vi "Open.vi"(8 "Error In":errorcluster, 10 "Enable Gestures? (T)":bool=TRUE) -> (0 "Error Out":errorcluster, 3 "Leap Handle":T1)   [LabVIEW 2014]
uses:
  Typedef 2.0/Leap Handle.ctl
  C:/Users/Frax/Desktop/Progetti avanzati Labview/Smart Wristband/Smart Wristband/Leap Motion VIs 2.0/LeapCSharp.NET4.0.dll
  LeapCSharp.NET4.0.dll
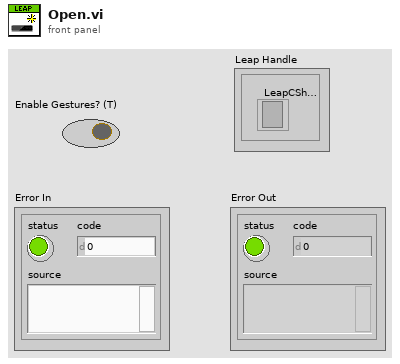
[diagram p1: front panel]
types:
  T1 = typedef "Leap Handle.ctl" = cluster{"LeapCSharp":refnum<k24>}
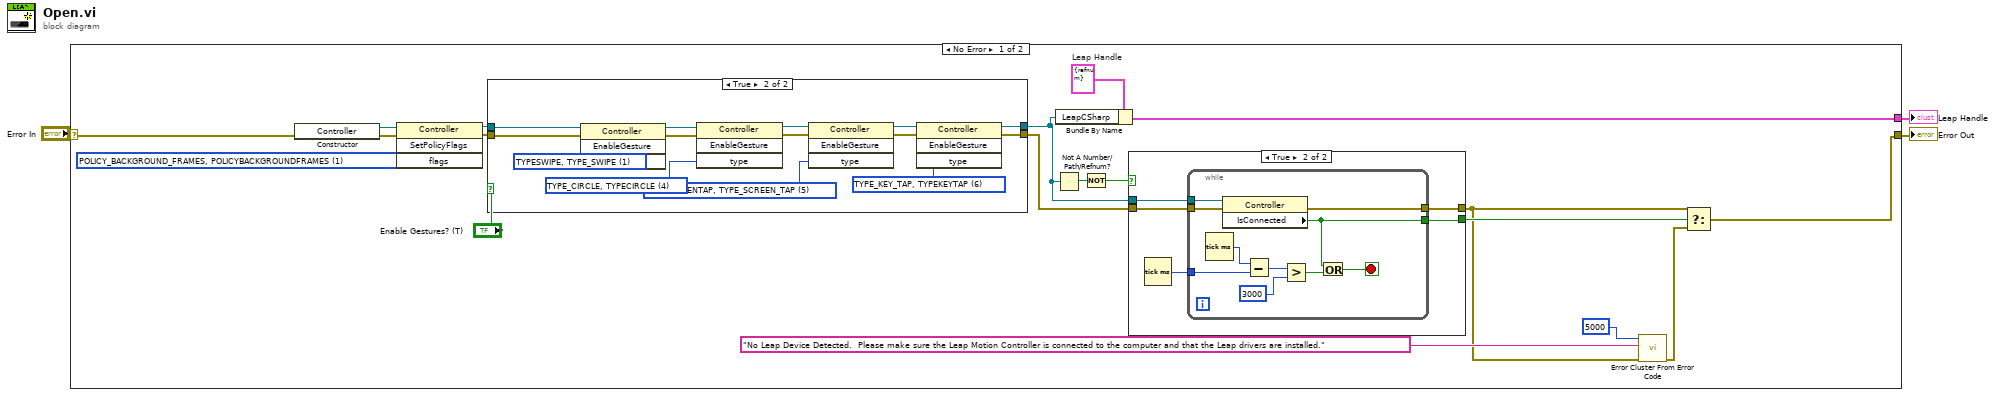
[diagram p0: block diagram]
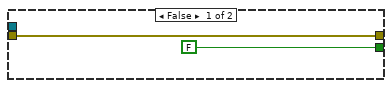
[diagram p2: hidden frame]
diagram:
  n1 = case shown="No Error" "Error In" {
    selector: "Error In" -> [w22 w56]
    tunnel: [w8 w56] -> w2
    tunnel: [w21 _] -> w1
    frame No Error {
      w5 = T1 {"LeapCSharp"=refnum}  # Leap Handle
      w6 = 1 items=["POLICYDEFAULT, POLICY_DEFAULT"=0, "POLICY_BACKGROUND_FRAMES, POLICYBACKGROUNDFRAMES"=1, "POLICY_IMAGES"=2, "POLICY_OPTIMIZE_HMD"=4] ("flags")
      n2 = constructor class="Controller"(error in=w22) -> (reference out=w16:refnum<k24>, error out=w19:errorcluster)  [unwired: 2 in, 1 out]
      n3 = invoke class="Controller" method="SetPolicyFlags"(reference=w16, error in=w19, "flags"=w6) -> (reference out=w17:refnum<k24>, error out=w18:errorcluster)  [unwired: 1 in, 2 out]
      n4 = case shown="True" "Enable Gestures? (T)" {
        tunnel: w17 -> [w40 w55]
        tunnel: w18 -> [w41 w54]
        tunnel: [w41 w53] -> w13
        tunnel: [w40 w52] -> w4
        frame False {
        }
        frame True {
          w42 = 6 items=["TYPESWIPE, TYPE_SWIPE"=1, "TYPE_CIRCLE, TYPECIRCLE"=4, "TYPESCREENTAP, TYPE_SCREEN_TAP"=5, "TYPE_KEY_TAP, TYPEKEYTAP"=6, "TYPE_INVALID, TYPEINVALID"=-1] ("type")
          w43 = 5 items=["TYPESWIPE, TYPE_SWIPE"=1, "TYPE_CIRCLE, TYPECIRCLE"=4, "TYPESCREENTAP, TYPE_SCREEN_TAP"=5, "TYPE_KEY_TAP, TYPEKEYTAP"=6, "TYPE_INVALID, TYPEINVALID"=-1] ("type")
          w44 = 4 items=["TYPESWIPE, TYPE_SWIPE"=1, "TYPE_CIRCLE, TYPECIRCLE"=4, "TYPESCREENTAP, TYPE_SCREEN_TAP"=5, "TYPE_KEY_TAP, TYPEKEYTAP"=6, "TYPE_INVALID, TYPEINVALID"=-1] ("type")
          w45 = 1 items=["TYPESWIPE, TYPE_SWIPE"=1, "TYPE_CIRCLE, TYPECIRCLE"=4, "TYPESCREENTAP, TYPE_SCREEN_TAP"=5, "TYPE_KEY_TAP, TYPEKEYTAP"=6, "TYPE_INVALID, TYPEINVALID"=-1] ("type")
          n5 = invoke class="Controller" method="EnableGesture"(reference=w55, error in=w54, "type"=w45) -> (reference out=w51:refnum<k24>, error out=w50:errorcluster)  [unwired: 1 in, 2 out]
          n6 = invoke class="Controller" method="EnableGesture"(reference=w51, error in=w50, "type"=w44) -> (reference out=w49:refnum<k24>, error out=w48:errorcluster)  [unwired: 1 in, 2 out]
          n7 = invoke class="Controller" method="EnableGesture"(reference=w49, error in=w48, "type"=w43) -> (reference out=w46:refnum<k24>, error out=w47:errorcluster)  [unwired: 1 in, 2 out]
          n8 = invoke class="Controller" method="EnableGesture"(reference=w46, error in=w47, "type"=w42) -> (reference out=w52:refnum<k24>, error out=w53:errorcluster)  [unwired: 1 in, 2 out]
        }
      }
      n9 = Bundle By Name(cluster=w5, "LeapCSharp"=w4) -> (w21:T1)
      n10 = Not A Number/Path/Refnum?(number/path/refnum=w4) -> (NaN/Path/Refnum?=w15:bool)
      n11 = Not(x=w15) -> (.not. x?=w14:bool)
      n12 = case shown="True" w14 {
        tunnel: w4 -> [_ w29]
        tunnel: w13 -> [w23 w28]
        tunnel: [FALSE ("IsConnected") w27] -> w12
        tunnel: [w23 w26] -> w7
        frame False {
        }
        frame True {
          n13 = Tick Count (ms)() -> (millisecond timer value=w25:u32)
          n14 = while {
            tunnel: w29 -> [w39]
            tunnel: w28 -> [w38]
            tunnel: [w31] -> w27
            tunnel: [w37] -> w26
            tunnel: w25 -> [w35]
            stop <- w30 stop-if-true
            n15 = Tick Count (ms)() -> (millisecond timer value=w36:u32)
            n16 = property class="Controller"(reference=w39, error in=w38) -> (error out=w37:errorcluster, "IsConnected"=w31:bool)  [unwired: 1 out]
            n17 = Subtract(x=w36, y=w35) -> (x-y=w34:u32)
            n18 = Greater?(x=w34, y=u32 3000) -> (0:w32:bool)
            n19 = Or(x=w31, y=w32) -> (x .or. y?=w30:bool)
          }
        }
      }
      n20 = call <vilib>:"Error Cluster From Error Code.vi"("error in (no error)"=w7, "error message (\"\")"="No Leap Device Detected.  Please make sure the Leap Motion Controller is connected to the computer and that the Leap drivers are installed." ("error message (\"\")"), "error code (0)"=5000) -> ("error out"=w9:errorcluster)  [unwired: 6 in]
      n21 = Select(t=w7, s=w12, f=w9) -> (s? t:f=w8:errorcluster)
    }
    frame Error {
    }
  }
  "Error Out" <- w2
  "Leap Handle" <- w1
